vi "test_Add Command_Use SysDef with Command with MetaData Channels.vi"(8 "error in (no error)":errorcluster, 11 "TestCase in":refnum<class "Instrument Addon Scripting API Messages Unit Tests.lvclass">) -> (0 "error out":errorcluster, 3 "TestCase out":refnum<class "Instrument Addon Scripting API Messages Unit Tests.lvclass">)   [LabVIEW 2019, in "Instrument Addon Scripting API Messages Unit Tests.lvclass"]
uses:
  Instrument Addon Scripting API Messages Unit Tests.lvclass
  APIs/Scripting API/TypeDefs/Command Settings.ctl
  <vilib>/NI VeriStand/Custom Device API/Custom Device Item Ref.ctl
  APIs/Scripting API/TypeDefs/Padding.ctl
  Addon/Addon Shared/Types/Command Parameters.ctl
  Addon/Addon Shared/Types/Linked Channel Cluster.ctl
  Addon/Addon Shared/Types/FG Control.ctl
  Instrument Addon Scripting API Messages Unit Tests.lvclass/Instrument Addon Scripting API Messages Unit Tests.ctl
  Addon/Addon Shared/SubVIs/Constants.vi
  <vilib>/NI/NI VeriStand Advanced SysDef API/_SubVIs/SysDef.Search.GUID.vi
  <vilib>/NI VeriStand/Custom Device API/NI VeriStand - Get Item Property.vi
  <vilib>/NI VeriStand/Custom Device API/Get Item Property (String).vi
  <vilib>/NI VeriStand/Custom Device API/Get Item Property (String Array).vi
  <vilib>/NI VeriStand/Custom Device API/Get Item Property (Boolean).vi
  <vilib>/NI VeriStand/Custom Device API/Get Item Property (U32).vi
  <vilib>/NI VeriStand/Custom Device API/NI VeriStand - Set Item Property.vi
  <vilib>/NI VeriStand/Custom Device API/Set Item Property (String).vi
  <vilib>/NI VeriStand/Custom Device API/Set Item Property (String Array).vi
  <vilib>/NI VeriStand/Custom Device API/Set Item Property (Boolean).vi
  <vilib>/NI VeriStand/Custom Device API/Set Item Property (U32).vi
  <vilib>/addons/_JKI Toolkits/VI Tester/TestCase.llb/TestCase.lvclass
  Instrument Addon Scripting API Test Assets/Instrument Addon Scripting API Test Assets.lvclass
  Addon/Addon Shared/Instrument Addon Shared.lvlib
  <vilib>/NI/NI VeriStand Advanced SysDef API/SysDef API/Advanced System Definition.lvlib
  <vilib>/NI VeriStand/Custom Device API/Custom Device API.lvlib
  APIs/Scripting API/Instrument Addon Scripting API.lvlib
  C:/Program Files (x86)/National Instruments/LabVIEW 2019/vi.lib/addons/_JKI Toolkits/VI Tester/TestCase.llb/TestCase.lvclass
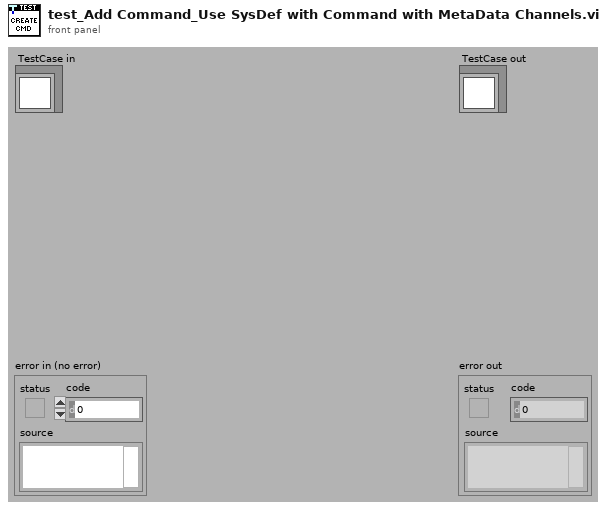
[diagram p1: front panel]
types:
  T1 = typedef "Instrument Addon Shared.lvlib/FG Control.ctl" = enum16{"Get", "Set"}
  T2 = typedef "Instrument Addon Scripting API.lvlib/Command Settings.ctl" = cluster{"Command Format":string, "Linked Channels":cluster{"Variable Name":string, "Channel Ref in":T3}[], "Use Padding?":bool, "Padding":T4}
  T3 = typedef "Custom Device API.lvlib/Custom Device Item Ref.ctl" = u64
  T4 = typedef "Instrument Addon Scripting API.lvlib/Padding.ctl" = cluster{"Pad Value":u8, "Length":u32}
  T5 = typedef "Instrument Addon Shared.lvlib/Command Parameters.ctl" = cluster{"Command":string, "Linked Channels":T6[], "Pad":bool, "Length":u32, "Pad Value":u8}
  T6 = typedef "Instrument Addon Shared.lvlib/Linked Channel Cluster.ctl" = cluster{"Variable Name":string, "GUID":string}
  T7 = typedef "Instrument Addon Scripting API.lvlib/Linked Channel.ctl" = cluster{"Variable Name":string, "Channel Refnum":T3}
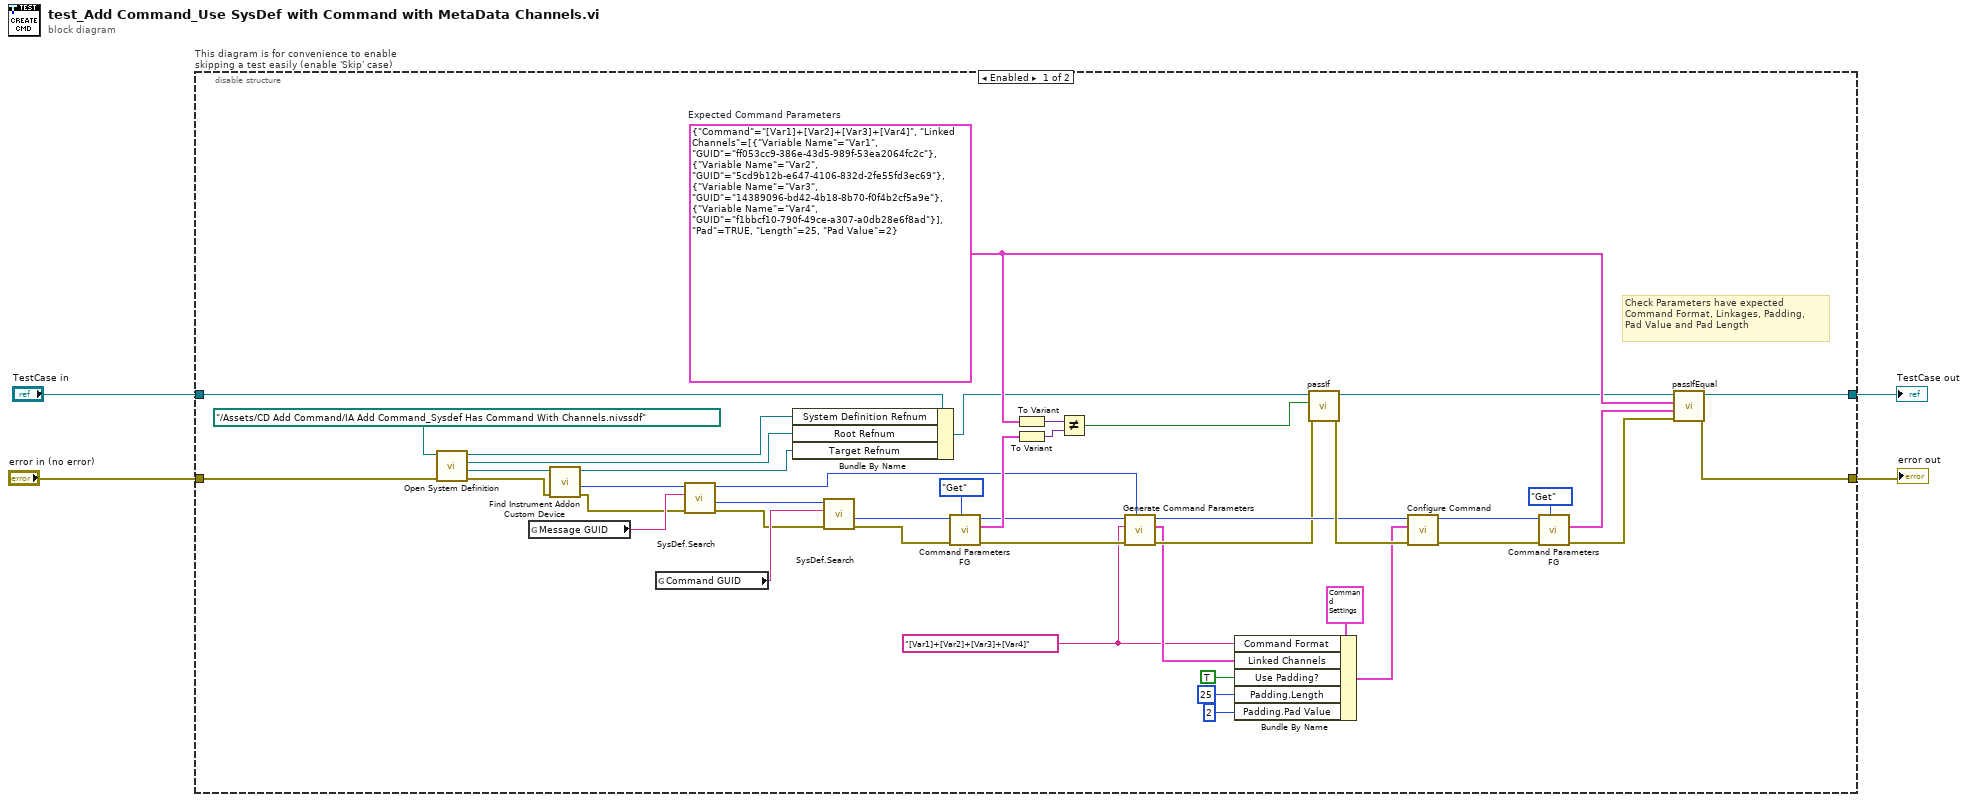
[diagram p0: block diagram]
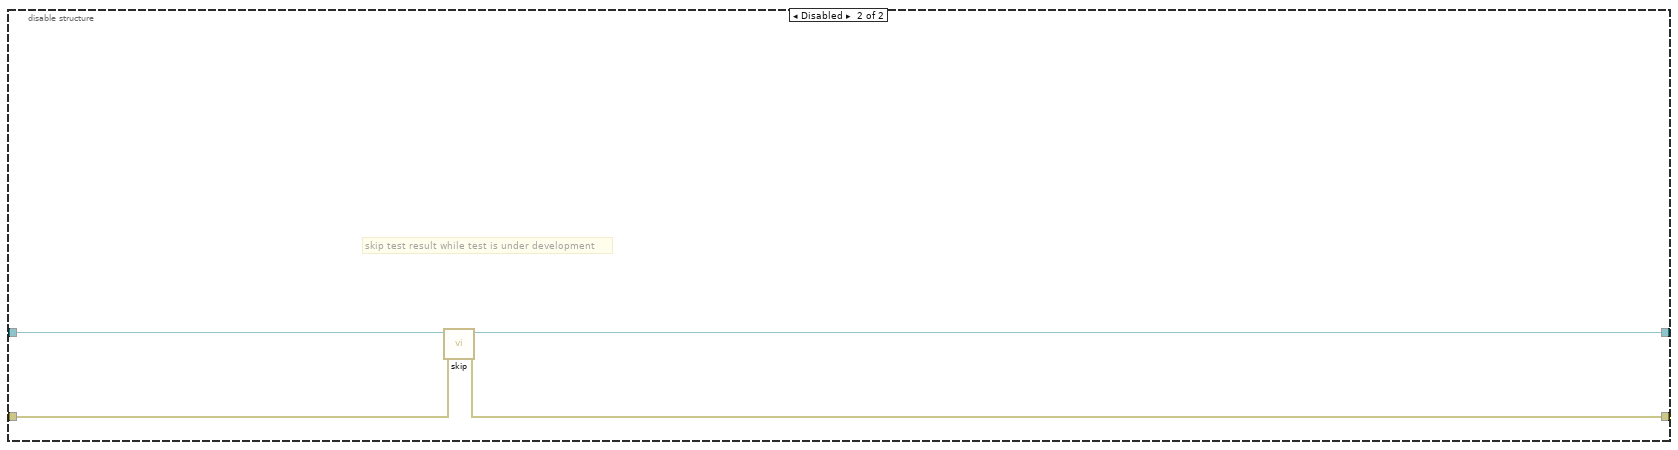
[diagram p2: hidden frame]
diagram:
  n1 = disable-structure "This diagram is for convenience to enable skipping a test easily (enable 'Skip' case)" shown="Enabled" {
    disable-tunnel: "TestCase in" -> [w22 w52]
    disable-tunnel: [w45 w50] -> w1
    disable-tunnel: [w46 w51] -> w3
    disable-tunnel: "error in (no error)" -> [w47 w49]
    frame Enabled {
      w24 = T5 {"Command"="[Var1]+[Var2]+[Var3]+[Var4]", "Linked Channels"=[{"Variable Name"="Var1", "GUID"="ff053cc9-386e-43d5-989f-53ea2064fc2c"}, {"Variable Name"="Var2", "GUID"="5cd9b12b-e647-4106-832d-2fe55fd3ec69"}, {"Variable Name"="Var3", "GUID"="14389096-bd42-4b18-8b70-f0f4b2cf5a9e"}, {"Variable Name"="Var4", "GUID"="f1bbcf10-790f-49ce-a307-a0db28e6f8ad"}], "Pad"=TRUE, "Length"=25, "Pad Value"=2}  # Expected Command Parameters
      w5 = "[Var1]+[Var2]+[Var3]+[Var4]" ("Command Format")
      # "Check Parameters have expected \nCommand Format, Linkages, Padding,\nPad Value and Pad Length"
      n2 = call "Open System Definition.vi"("error in (no error)"=w47, "System Definition File"=path "../Assets/CD Add Command/IA Add Command_Sysdef Has Command With Channels.nivssdf" ("SDF file")) -> ("error out"=w40:errorcluster, "Target Refnum"=w41:refnum<k24>, "Root Refnum"=w19:refnum<k24>, "System Definition Refnum"=w20:refnum<k24>)  [unwired: 6 in]
      n3 = global read "Constants.vi" "Message GUID"() -> (w39:string)
      n4 = call "Find Instrument Addon Custom Device.vi"("error in"=w40, "target in"=w41) -> ("error out"=w12:errorcluster, "NodeID"=w13:u64, "target out"=w18:refnum<k24>)  [unwired: 7 in]
      n5 = global read "Constants.vi" "Command GUID"() -> (w34:string)
      n6 = call-poly <vilib>:"SysDef.Search.vi"("error in (no error)"=w12, "GUID"=w39, "nodeID"=w13) -> ("error out"=w29:errorcluster, "Value out"=w30:u64, "nodeID out"=w7:u64)  [unwired: 5 in, 1 out]
      n7 = Bundle By Name(cluster=w22, "System Definition Refnum"=w20, "Root Refnum"=w19, "Target Refnum"=w18) -> (w21:refnum<class "Instrument Addon Scripting API Messages Unit Tests.lvclass">)
      n8 = call-poly <vilib>:"SysDef.Search.vi"("error in (no error)"=w29, "GUID"=w34, "nodeID"=w30) -> ("error out"=w32:errorcluster, "Value out"=w33:u64)  [unwired: 5 in, 2 out]
      n9 = call "Command Parameters FG.vi"("Action"=FG_Control."Get", "error in (no error)"=w32, "Item Ref in"=w33) -> ("error out"=w9:errorcluster, "Command Parameters"=w25:T5, "Item Ref out"=w11:T3)  [unwired: 6 in]
      n10 = To Variant(anything=w24) -> (Variant=w28:variant)
      n11 = To Variant(anything=w25) -> (Variant=w27:variant)
      n12 = Not Equal?(x=w28, y=w27) -> (x != y?=w26:bool)
      n13 = call "Generate Command Parameters.vi"("Instrument Addon Refnum in"=w7, "Error In"=w9, "Command String"=w5, "Command Channel in"=w11) -> ("Error Out"=w8:errorcluster, "Linked Channels"=w6:T7[], "Command Channel out"=w10:T3)  [unwired: 4 in, 1 out]
      n14 = Bundle By Name(cluster=T2 {"Command Format"="[Var1]+[Var2]", "Linked Channels"=[{"Variable Name"="Var1", "Channel Ref in"=32}, {"Variable Name"="Var2", "Channel Ref in"=33}], "Use Padding?"=FALSE, "Padding"={"Pad Value"=0, "Length"=0}} ("Settings"), "Command Format"=w5, "Linked Channels"=w6, "Use Padding?"=TRUE ("Pad"), "Padding.Length"=u32 25, "Padding.Pad Value"=u8 2) -> (w14:T2)
      n15 = call-dynamic "passIf.vi"("error in (no error)"=w8, "pass"=w26, "TestCase in"=w21) -> ("error out"=w17:errorcluster, "TestCase out"=w23:refnum<class "Instrument Addon Scripting API Messages Unit Tests.lvclass">)  [unwired: 7 in]
      n16 = call "Configure Command.vi"("error in (no error)"=w17, "settings"=w14, "command refnum in"=w10) -> ("error out"=w16:errorcluster, "command refnum out"=w15:T3)  [unwired: 7 in]
      n17 = call "Command Parameters FG.vi"("Action"=FG_Control."Get", "error in (no error)"=w16, "Item Ref in"=w15) -> ("error out"=w43:errorcluster, "Command Parameters"=w42:T5)  [unwired: 6 in, 1 out]
      n18 = call-dynamic "passIfEqual.vi"("error in (no error)"=w43, "y"=w42, "x"=w24, "TestCase in"=w23) -> ("error out"=w46:errorcluster, "TestCase out"=w45:refnum<class "Instrument Addon Scripting API Messages Unit Tests.lvclass">)  [unwired: 6 in]
    }
    frame Disabled {
      # "skip test result while test is under development"
      n19 = call <vilib>:"skip.vi"("error in (no error)"=w49, "TestCase in"=w52) -> ("error out"=w51:errorcluster, "TestCase out"=w50:refnum<class "Instrument Addon Scripting API Messages Unit Tests.lvclass">)  [unwired: 8 in]
    }
  }
  "error out" <- w3
  "TestCase out" <- w1
